vi "Lake Shore 325 Configure Control Parameters and Aquire Single Readiing.vi"(0 "VISA resource name":refnum<visa-resource-name>, 5 "Input (0:A)":u16(ring) items=["A", "B"]) -> ()   [LabVIEW 2019]
doc: "This VI was designed to demonstrate typical usage of sub VIs containing the more common 325 functions. The VI Initializes the instrument, allows the user to determine if control parameters and setpoint values are sent, takes a single sensor reading, reads the heater output value, and then closes the instrument."
uses:
  Public/Data/Sensor Data (Single Reading).vi
  Lake Shore 325.lvlib
panel:
  in  "Mode (1:Manual PID)":u16(ring)=1 items=["Manual PID"=1, "Zone"=2, "Open Loop"=3, "AutoTune PID"=4, "AutoTune PI"=5, "AutoTune P"=6]
  in  "Set Setpoint (F: Don't Set)":bool
  in  "Setpoint Value (0.0000)":dbl format="%.4f"
  in  "Heater Resistance (1:25 Ohm)":u16(ring)=1 items=["25 Ohm"=1, "50 Ohm"=2]
  in  "Manual Heater Power (0.000 %)":dbl format="%.3f"
  in  "Rate (D) (0 %)":u16
  in  "Reset (I) (0.0)":dbl format="%.1f"
  in  "Gain (P) (0.0)":dbl format="%.1f"
  in  "Heater Range (0:Off)":u16(ring) items=["Off", "Low (loop 1) or On (loop 2)", "High (loop 1)"]
  in  "Control Input (0:A)":u16(ring) items=["A", "B"]
  in  "Setpoint Units (1:Kelvin)":u16(ring)=1 items=["Kelvin"=1, "Celsius"=2, "Sensor Units"=3]
  out "Heater Output Value (0.0 %)":dbl format="%.1f"
  in  "Loop (1:Loop 1)":u16(ring)=1 items=["Loop 1"=1, "Loop 2"=2]
  in  "Data Source (0:Kelvin)":u16(ring) items=["Kelvin", "Celsius", "Sensor Units"]
  out "Sensor Data (0.0000)":dbl format="%.4f"
  in  "Serial Configuration":T1={"Baud Rate"=9600, "Parity"=1, "Data Bits"=7, "Stop Bits"=10, "Flow Control"=0} {"Flow Control" items=["None", "XON/XOFF", "RTS/CTS", "XON/XOFF & RTS/CTS", "DTR/DSR", "XON/XOFF & DTR/DSR"]; "Stop Bits" items=["1.0"=10, "1.5"=15, "2.0"=20]; "Data Bits" items=["7"=7, "8"=8]; "Parity" items=["None", "Odd", "Even", "Mark", "Space"]; "Baud Rate" items=["300"=300, "600"=600, "1200"=1200, "2400"=2400, "4800"=4800, "9600"=9600, "19200"=19200, "38400"=38400, "57600"=57600]}
  in  "Configure Control Parameters (F: Don't Configure)":bool
  # "© 2006 Lake Shore Cryotronics Inc.  ALL RIGHTS RESERVED."
  # "Control Parameters"
  # "Sensor Data"
  # "Setpoint"
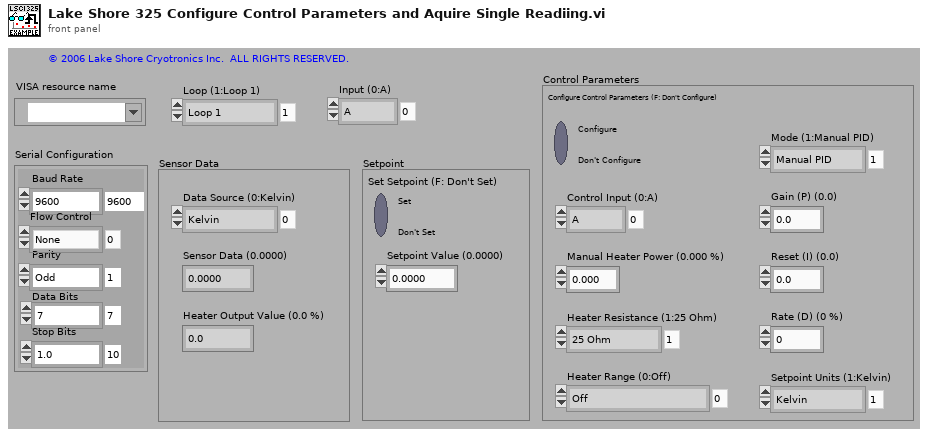
[diagram p1: front panel]
types:
  T1 = cluster{"Baud Rate":u32, "Parity":u16, "Data Bits":u16, "Stop Bits":u16, "Flow Control":u16}
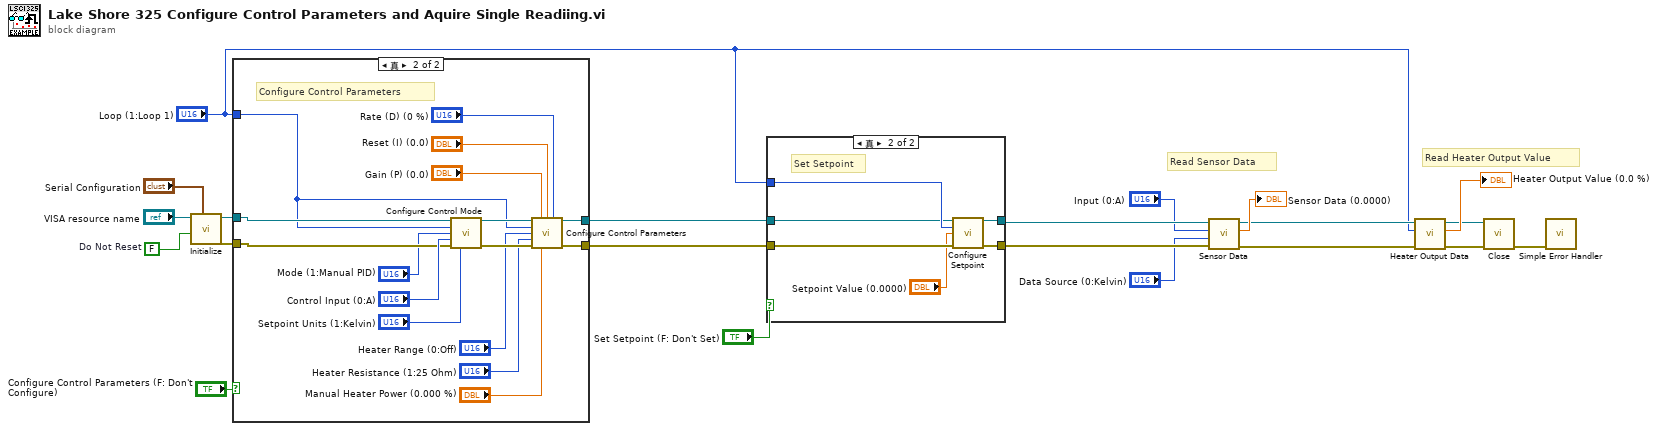
[diagram p0: block diagram]
diagram:
  w1 = FALSE  # Do Not Reset
  # "Read Heater Output Value"
  # "Read Sensor Data"
  n1 = call "Initialize.vi"("Serial Configuration"="Serial Configuration", "Reset (True)"=w1, "VISA resource name"="VISA resource name") -> ("error out"=w20:errorcluster, "VISA resource name out"=w21:refnum<visa-resource-name>)  [unwired: 7 in]
  n2 = case shown="真" "Configure Control Parameters (F: Don't Configure)" {
    tunnel: "Loop (1:Loop 1)" -> [_ w30]
    tunnel: w21 -> [w23 w32]
    tunnel: w20 -> [w22 w31]
    tunnel: [w22 w26] -> w2
    tunnel: [w23 w25] -> w3
    frame False {
      # "Do Not Configure Control Parameters"
    }
    frame True {
      # "Configure Control Parameters"
      n3 = call "Configure Control Mode.vi"("VISA resource name"=w32, "Loop (1:Loop 1)"=w30, "Mode (1:Manual PID)"="Mode (1:Manual PID)", "Control Input (0:A)"="Control Input (0:A)", "error in (no error)"=w31, "Setpoint Units (1:Kelvin)"="Setpoint Units (1:Kelvin)") -> ("VISA resource name out"=w34:refnum<visa-resource-name>, "error out"=w33:errorcluster)  [unwired: 8 in]
      n4 = call "Configure Control Parameters.vi"("VISA resource name"=w34, "Gain (P) (0.0)"="Gain (P) (0.0)", "Reset (I) (0.0)"="Reset (I) (0.0)", "Rate (D) (0 %)"="Rate (D) (0 %)", "Loop (1:Loop 1)"=w30, "Heater Range (0:Off)"="Heater Range (0:Off)", "Heater Resistance (1:25 Ohm)"="Heater Resistance (1:25 Ohm)", "error in (no error)"=w33, "Manual Heater Power (0.000 %)"="Manual Heater Power (0.000 %)") -> ("VISA resource name out"=w25:refnum<visa-resource-name>, "error out"=w26:errorcluster)  [unwired: 5 in]
    }
  }
  n5 = case shown="真" "Set Setpoint (F: Don't Set)" {
    tunnel: "Loop (1:Loop 1)" -> [_ w47]
    tunnel: w3 -> [w41 w46]
    tunnel: w2 -> [w40 w45]
    tunnel: [w40 w43] -> w16
    tunnel: [w41 w42] -> w17
    frame False {
      # "Do Not Set Setpoint"
    }
    frame True {
      # "Set Setpoint"
      n6 = call "Configure Setpoint.vi"("VISA resource name"=w46, "Loop (1:Loop 1)"=w47, "Setpoint Value (0.0000)"="Setpoint Value (0.0000)", "error in (no error)"=w45) -> ("VISA resource name out"=w42:refnum<visa-resource-name>, "error out"=w43:errorcluster)  [unwired: 10 in]
    }
  }
  n7 = call-poly "Sensor Data.vi"("error in (no error)"=w16, "Data Source (0:Kelvin)"="Data Source (0:Kelvin)", "Sensor Input (0:A)"="Input (0:A)", "VISA resource name"=w17) -> ("error out"=w11:errorcluster, "Sensor Data"=→"Sensor Data (0.0000)":dbl, "VISA resource name out"=w12:refnum<visa-resource-name>)  [unwired: 5 in]
  n8 = call "Heater Output Data.vi"("error in (no error)"=w11, "Loop (1:Loop 1)"="Loop (1:Loop 1)", "VISA resource name"=w12) -> ("error out"=w7:errorcluster, "Heater Output Value"=→"Heater Output Value (0.0 %)":dbl, "VISA resource name out"=w8:refnum<visa-resource-name>)  [unwired: 6 in]
  n9 = call "Close.vi"("error in (no error)"=w7, "VISA resource name"=w8) -> ("error out"=w4:errorcluster)  [unwired: 9 in]
  n10 = call <vilib>:"Simple Error Handler.vi"("error in (no error)"=w4) -> ()  [unwired: 4 in, 5 out]
